vi "Thermometer_Example.vi"() -> ()   [LabVIEW 2011]
uses:
  Root_XControl/Root_XControl.xctl
panel:
  in  "# Controls":i32=2
  in  "stop":bool
  out "Root_XControl":dbl[](xcontrol)
  # "Press Run to start this example. Change the number of controls to view. This increases\nor decreases the size of a random array of numbers. New controls\nwill automatically be instantiated to begin reflecting the new values. If the size decreases,\nthe extra controls will be stopped and removed automatically. When you press Stop,\nall controls are stopped and removed."
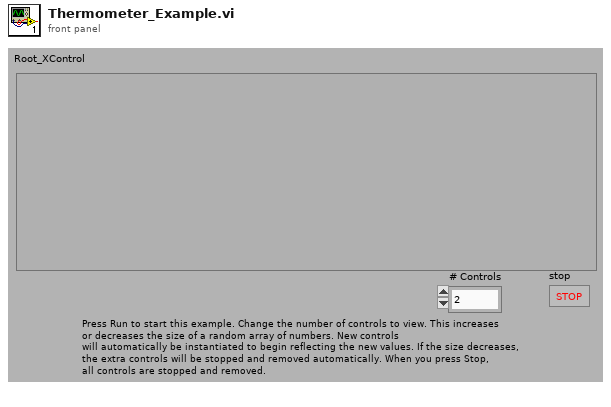
[diagram p1: front panel]
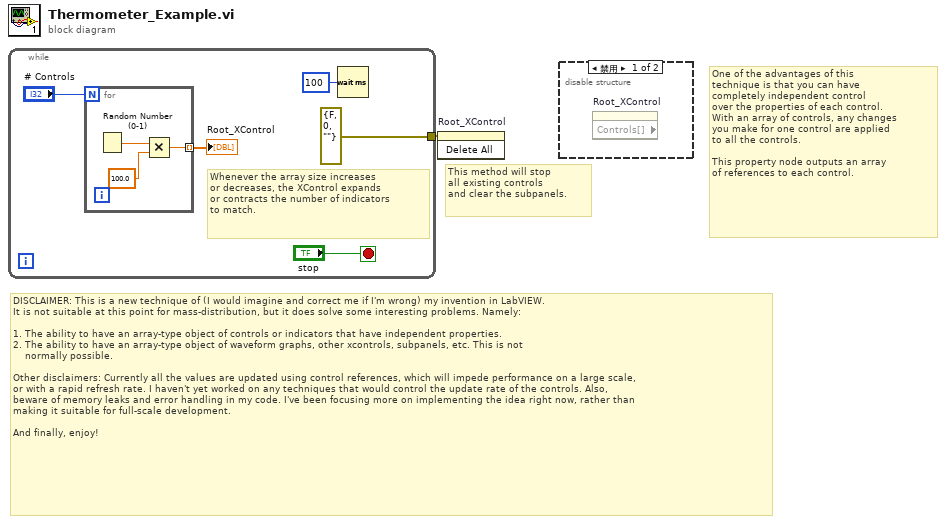
[diagram p0: block diagram]
diagram:
  # "This method will stop\nall existing controls\nand clear the subpanels."
  # "DISCLAIMER: This is a new technique of (I would imagine and correct me if I'm wrong) my invention in LabVIEW.\nIt is not suitable at this point for mass-distribution, but it does solve some interesting problems. Namely:\n\n1. The ability to have an array-type object of controls or indicators that have independent properties.\n2. The ability to have an array-type object of waveform graphs, other xcontrols, subpanels, etc. This is not\n    normally possible.\n\nOther disclaimers: Currently all the values are updated using control references, which will impede performance on a large scale,\nor with a rapid refresh rate. I haven't yet worked on any techniques that would control the update rate of the controls. Also,\nbeware of memory leaks and error handling in my code. I've been focusing more on implementing the idea right now, rather than\nmaking it suitable for full-scale development.\n\nAnd finally, enjoy!"
  # "One of the advantages of this\ntechnique is that you can have\ncompletely independent control\nover the properties of each control.\nWith an array of controls, any changes\nyou make for one control are applied\nto all the controls.\n\nThis property node outputs an array\nof references to each control."
  n1 = while {
    tunnel: [errorcluster {"status"=FALSE, "code"=0, "source"=""} ("error in 2 (no error)")] -> w1
    stop <- "stop" stop-if-true
    # "Whenever the array size increases\nor decreases, the XControl expands\nor contracts the number of indicators\nto match."
    n2 = for {
      N: "# Controls" -> [_]
      tunnel: [w7] -> w3 mode=indexing
      n3 = Random Number (0-1)() -> (number: 0 to 1=w9:dbl)
      n4 = Multiply(x=w9, y=100.0) -> (x*y=w7:dbl)
    }
    "Root_XControl" <- w3
    n5 = Wait (ms)(milliseconds to wait=u32 100) -> ()  [unwired: 1 out]
  }
  n6 = invoke on="Root_XControl" class="Root_XControl (strict)" method="Delete All"(error in=w1) -> ()  [unwired: 2 in, 3 out]
  n7 = disable-structure shown="禁用" {
    frame Disabled {
      n8 = property on="Root_XControl" class="Root_XControl (严格)" props=["Controls[]"]() -> ()  [unwired: 2 in, 3 out]
    }
    frame Enabled {
    }
  }
